vi "EdgeChange_Example.vi"() -> ()   [LabVIEW 2019]
uses:
  <vilib>/Rock Robotics/WPI/ThirdParty/JAS_Junk/TrajLib/VI/Util_GetTime_U32.vi
  <vilib>/Rock Robotics/WPI/ThirdParty/JAS_Junk/TrajLib/Timer_New.vi
  <vilib>/Rock Robotics/WPI/ThirdParty/JAS_Junk/TrajLib/VI/TimeInterpBoolean_New.vi
  <vilib>/Rock Robotics/WPI/ThirdParty/JAS_Junk/TrajLib/VI/TimeInterpBoolean_AddSample.vi
  <vilib>/Rock Robotics/WPI/ThirdParty/JAS_Junk/TrajLib/VI/TimeInterpBoolean_GetSample.vi
  <vilib>/Rock Robotics/WPI/ThirdParty/JAS_Junk/TrajLib/VI/TimeInterpBoolean_SetMaxTime.vi
  <vilib>/Rock Robotics/WPI/ThirdParty/JAS_Junk/TrajLib/VI/TimeInterpBoolean_CleanUp.vi
  <vilib>/Rock Robotics/WPI/ThirdParty/JAS_Junk/TrajLib/VI/Util_GetTime_U64.vi
  <vilib>/Utility/semaphor.llb/Obtain Semaphore Reference.vi
  <vilib>/Rock Robotics/WPI/ThirdParty/JAS_Junk/TrajLib/Timer_Reset.vi
  <vilib>/Rock Robotics/WPI/ThirdParty/JAS_Junk/TrajLib/Timer_Start.vi
  <vilib>/Rock Robotics/WPI/ThirdParty/JAS_Junk/TrajLib/Timer_HasPeriodPassedOnce.vi
  <vilib>/gmath/interp.llb/Search Ordered Table.vi
  <vilib>/Rock Robotics/WPI/ThirdParty/JAS_Junk/TrajLib/Trajectory_Library.lvlib
panel:
  in  "Input":bool
  out "Edge Off":bool
  out "Edge Change":bool
  out "Waveform Chart":cluster{i16, i16, i16, i16}(graph)
  out "Edge On":bool
  out "Input":bool
  # "EDGE CHANGE EXAMPLE"
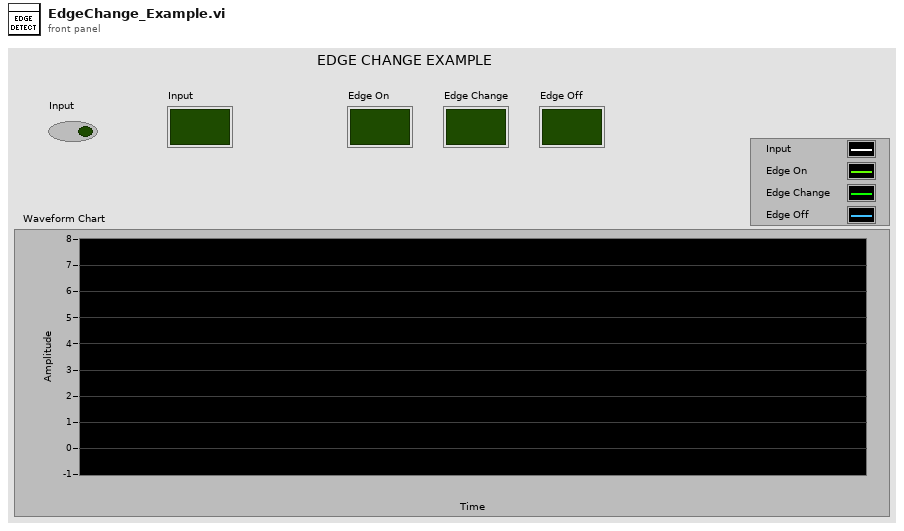
[diagram p1: front panel]
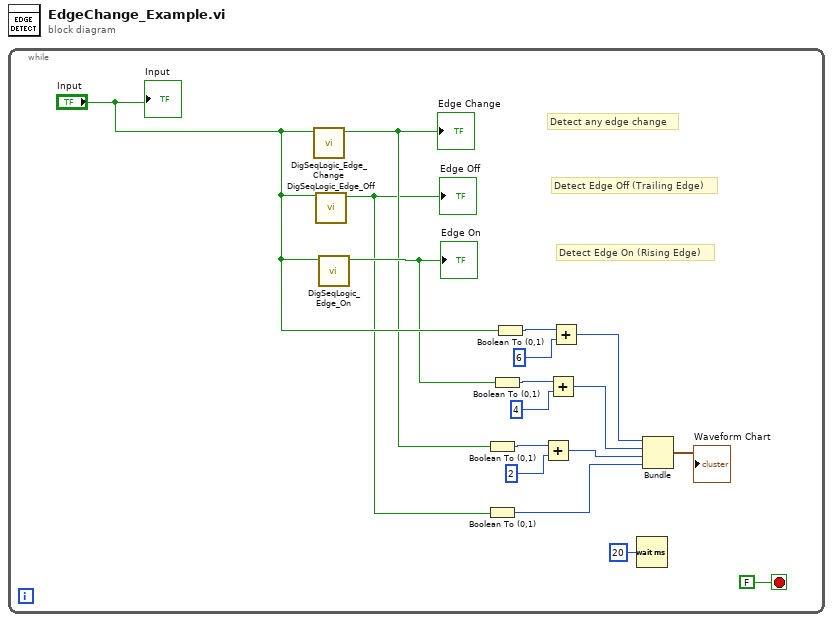
[diagram p0: block diagram]
diagram:
  n1 = while {
    stop <- FALSE stop-if-true
    # "Detect Edge On (Rising Edge)"
    # "Detect Edge Off (Trailing Edge)"
    # "Detect any edge change"
    n2 = call <vilib>:"DigSeqLogic_Edge_Change.vi"("Input"="Input") -> ("Any Edge"=w2:bool)  [unwired: 10 in]
    "Edge Change" <- w2
    n3 = call <vilib>:"DigSeqLogic_Edge_Off.vi"("Input"="Input") -> ("Off Edge"=w1:bool)  [unwired: 10 in]
    "Edge Off" <- w1
    n4 = call <vilib>:"DigSeqLogic_Edge_On.vi"("Input"="Input") -> ("On Edge"=w3:bool)  [unwired: 10 in]
    "Edge On" <- w3
    n5 = Boolean To (0,1)(Boolean=w2) -> (0, 1=w13:i16)
    n6 = Boolean To (0,1)(Boolean=w1) -> (0, 1=w11:i16)
    n7 = Boolean To (0,1)(Boolean=w3) -> (0, 1=w9:i16)
    n8 = Boolean To (0,1)(Boolean="Input") -> (0, 1=w7:i16)
    n9 = Add(x=w13, y=i16 2) -> (x+y=w12:i16)
    n10 = Add(x=w9, y=i16 4) -> (x+y=w6:i16)
    n11 = Add(x=w7, y=i16 6) -> (x+y=w5:i16)
    n12 = Wait (ms)(milliseconds to wait=u32 20) -> ()  [unwired: 1 out]
    n13 = Bundle(w5, w6, w12, w11) -> (→"Waveform Chart":cluster{i16, i16, i16, i16})  [unwired: 1 in]
    "Input" <- "Input"
  }
